vi "Mini_Test_App.vi"() -> ()   [LabVIEW 2015]
uses:
  Type Definitions/Mini_Test_App_Data.ctl
  <vilib>/Utility/error.llb/DialogType.ctl
panel:
  out "HP FAIL":bool
  out "HP PASS":bool
  out "HP UT":bool
  in  "Stop Hi-Pot":bool
  in  "Start Hi-Pot":bool
  out "GB FAIL":bool
  out "GB PASS":bool
  out "GB UT":bool
  in  "Stop GB":bool
  in  "Start GB":bool
  in  "Exit":bool
  # "Interface type: NI USB-6525"
  # "Warning. This app is a proof of concept and has no other purpose, \nit is not intended for production. Likewise, it has no error handling. \nUse at your own risk."
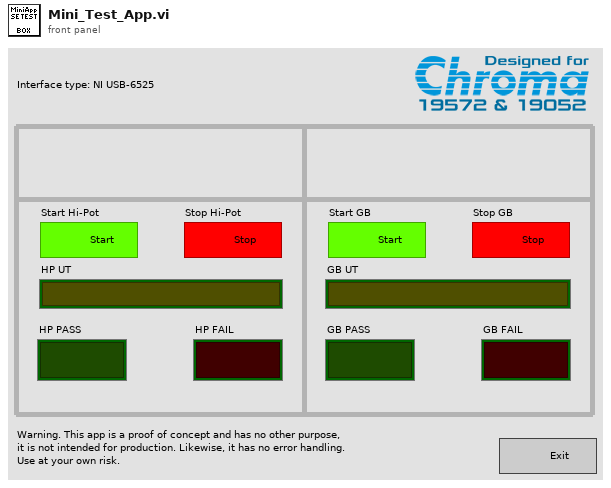
[diagram p1: front panel]
types:
  T1 = typedef "DialogType.ctl" = u16
  T2 = typedef "Mini_Test_App_Data.ctl" = cluster{"GB states":cluster{"UT":bool, "PASS":bool, "FAIL":bool}, "HP states":cluster{"UT":bool, "PASS":bool, "FAIL":bool}}
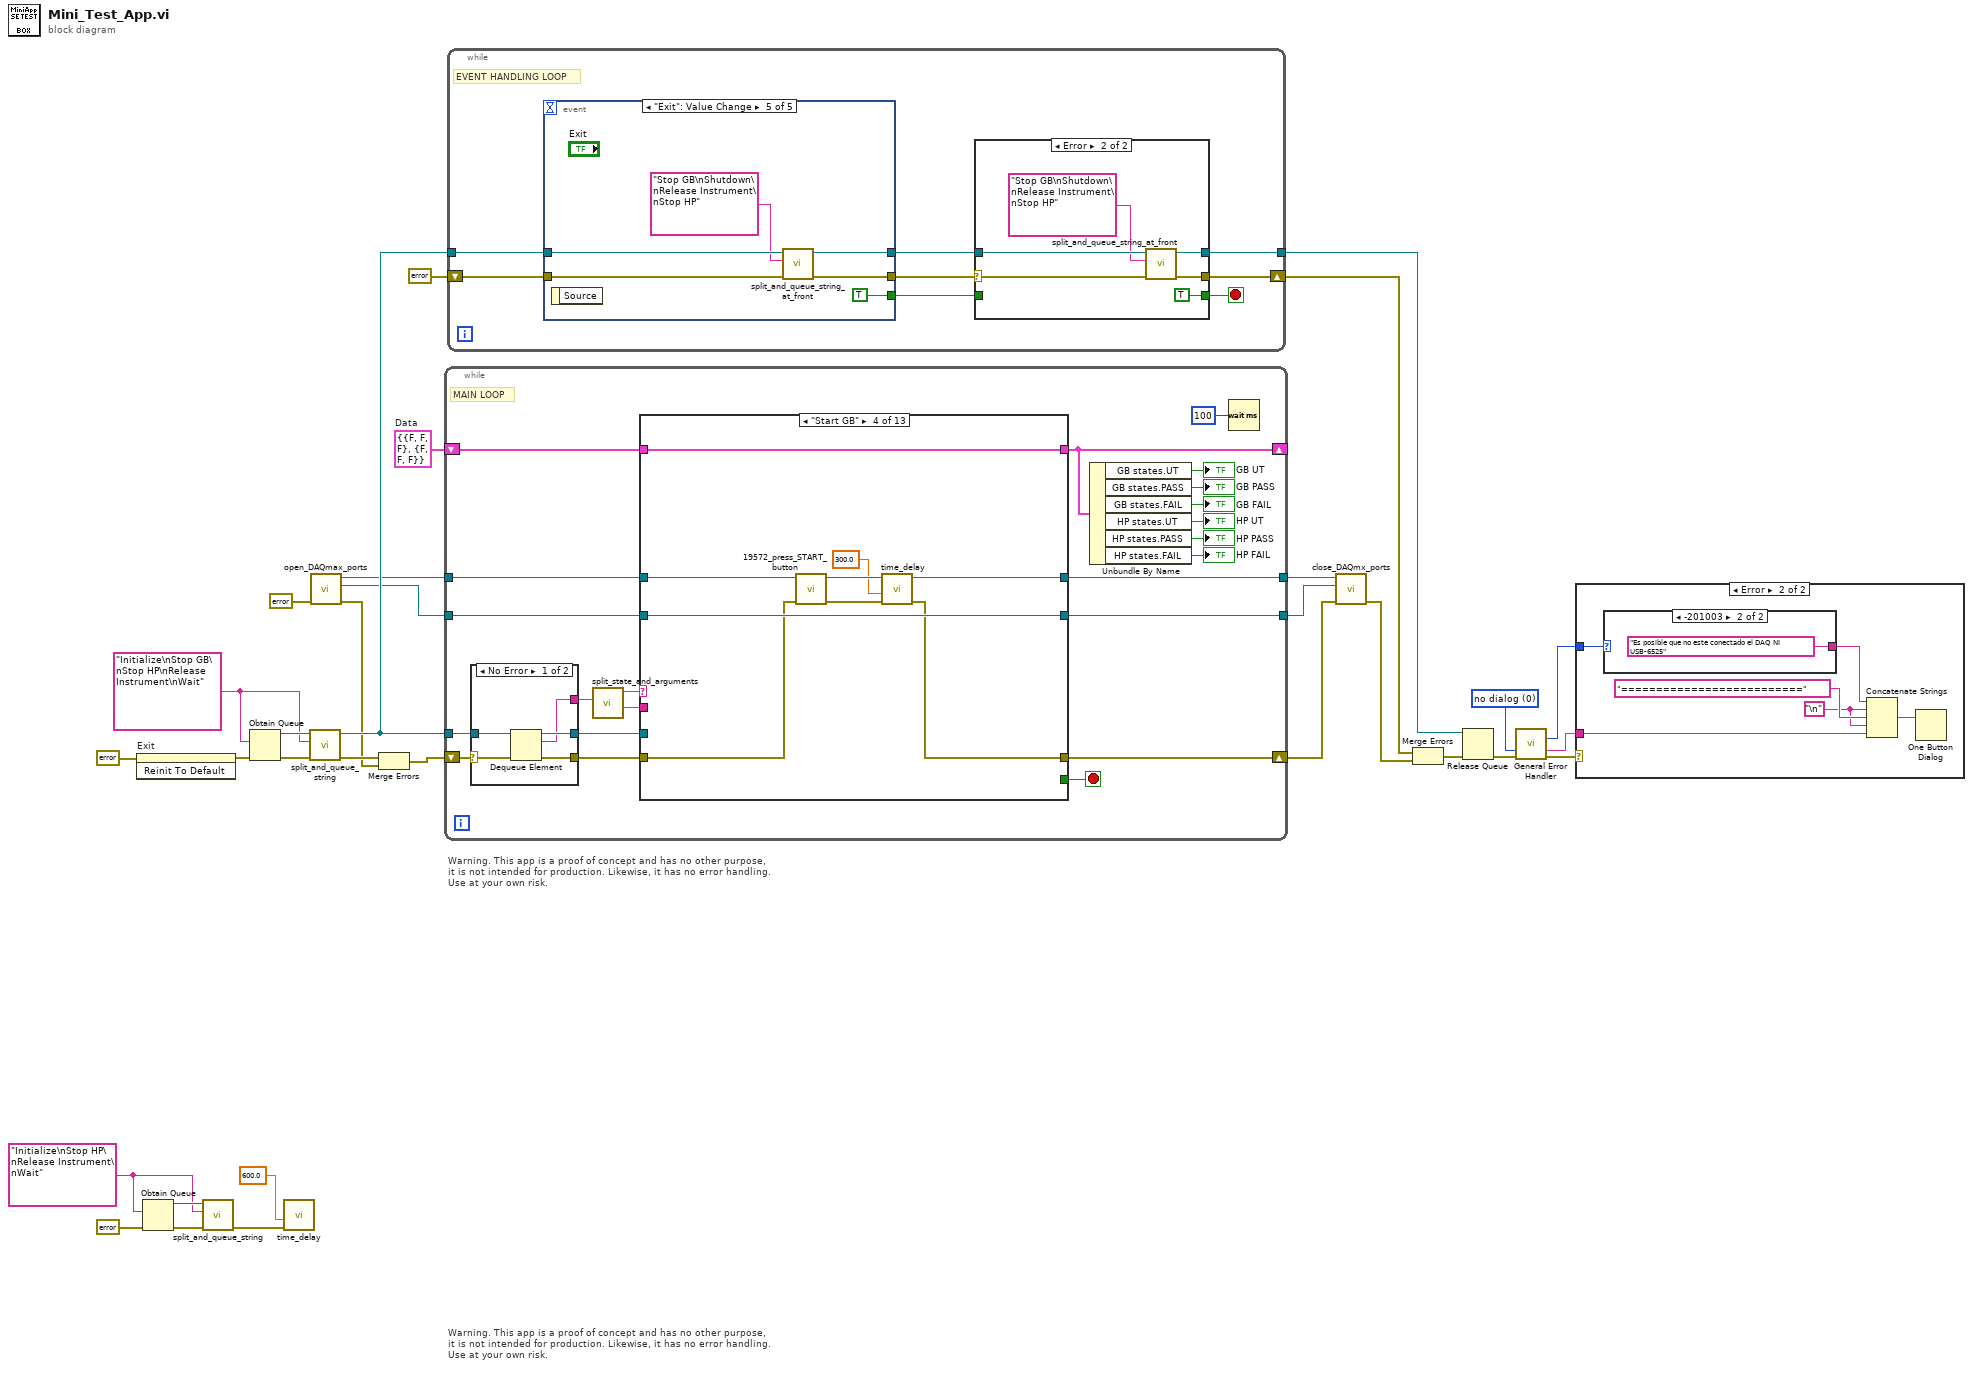
[diagram p0: block diagram]
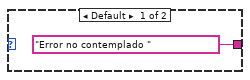
[diagram p3: hidden frame]
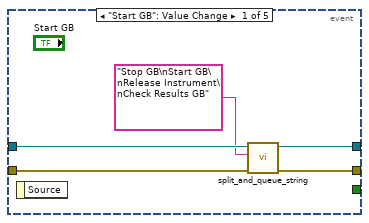
[diagram p5: hidden frame]
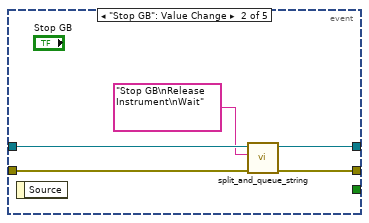
[diagram p6: hidden frame]
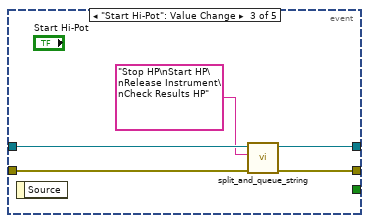
[diagram p7: hidden frame]
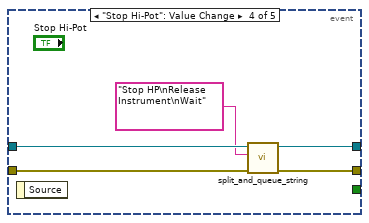
[diagram p8: hidden frame]
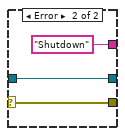
[diagram p9: hidden frame]
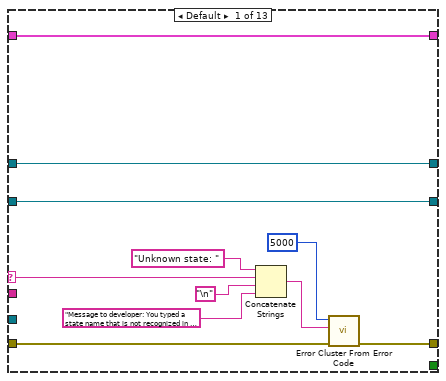
[diagram p10: hidden frame]
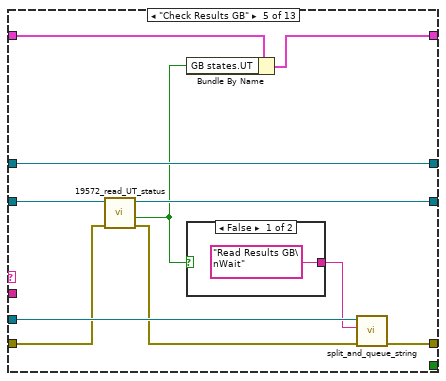
[diagram p13: hidden frame]
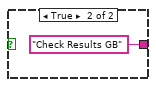
[diagram p14: hidden frame]
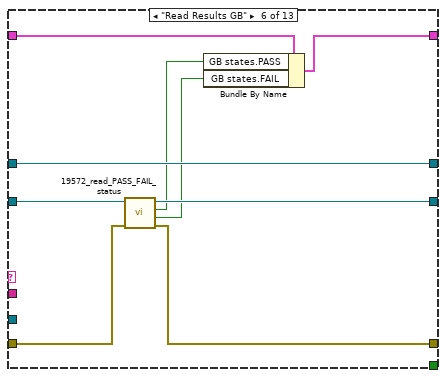
[diagram p15: hidden frame]
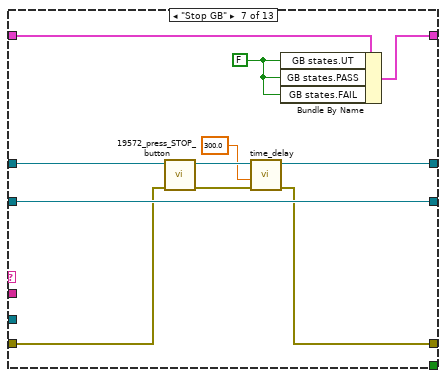
[diagram p16: hidden frame]
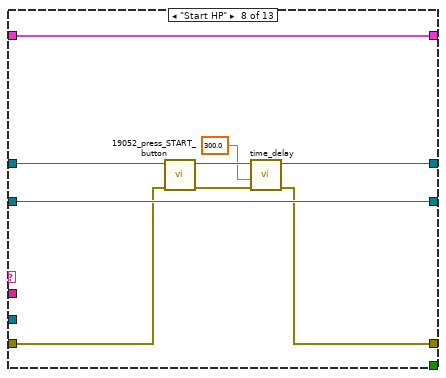
[diagram p17: hidden frame]
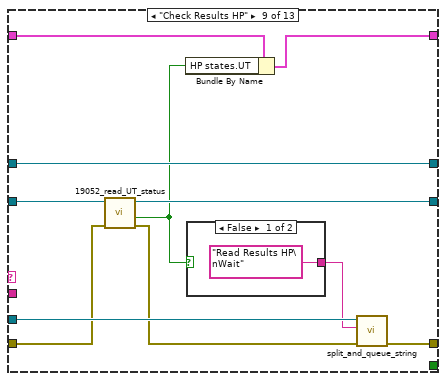
[diagram p18: hidden frame]
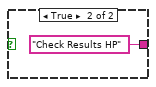
[diagram p19: hidden frame]
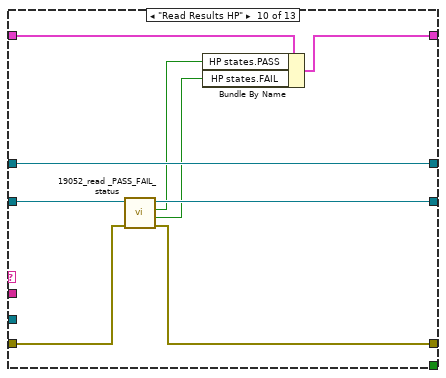
[diagram p20: hidden frame]
diagram:
  w1 = T1 0 items=["no dialog", "OK message", "continue or stop message", "OK message + warnings", "continue/stop + warnings"] ("type of dialog (OK msg:1)")
  w11 = "Initialize\nStop HP\nRelease Instrument\nWait"
  w20 = T2 {"GB states"={"UT"=FALSE, "PASS"=FALSE, "FAIL"=FALSE}, "HP states"={"UT"=FALSE, "PASS"=FALSE, "FAIL"=FALSE}}  # Data
  w22 = "Initialize\nStop GB\nStop HP\nRelease Instrument\nWait"
  # "Warning. This app is a proof of concept and has no other purpose, \nit is not intended for production. Likewise, it has no error handling. \nUse at your own risk."
  # "Warning. This app is a proof of concept and has no other purpose, \nit is not intended for production. Likewise, it has no error handling. \nUse at your own risk."
  n1 = invoke on="Exit" class="Bool (strict)" method="Reinit To Default"(error in=errorcluster {"status"=FALSE, "code"=0, "source"=""} ("error constant")) -> (error out=w17:errorcluster)  [unwired: 2 in, 2 out]
  n2 = Obtain Queue(element data type=w11, error in (no error)=errorcluster {"status"=FALSE, "code"=0, "source"=""} ("error constant")) -> (queue out=w13:refnum<queue>, error out=w12:errorcluster)  [unwired: 3 in, 1 out]
  n3 = call "split_and_queue_string.vi"("error in (no error)"=w12, "program string"=w11, "queue in"=w13) -> ("error out"=w7:errorcluster)  [unwired: 7 in, 1 out]
  n4 = Obtain Queue(element data type=w22, error in (no error)=w17) -> (queue out=w26:refnum<queue>, error out=w28:errorcluster)  [unwired: 3 in, 1 out]
  n5 = call "time_delay.vi"("error in (no error)"=w7, "milliseconds to wait"=600.0) -> ()  [unwired: 9 in, 1 out]
  n6 = call "split_and_queue_string.vi"("error in (no error)"=w28, "program string"=w22, "queue in"=w26) -> ("error out"=w27:errorcluster, "queue out"=w32:refnum<queue>)  [unwired: 7 in]
  n7 = call "open_DAQmax_ports.vi"("error in (no error)"=errorcluster {"status"=FALSE, "code"=0, "source"=""} ("error constant")) -> ("error out"=w21:errorcluster, "UT/PASS/FAIL states out"=w14:refnum<k21>, "START/STOP buttons out"=w15:refnum<k21>)  [unwired: 8 in]
  n8 = Merge Errors(w27, w21) -> (w16:errorcluster)
  n9 = while {
    tunnel: w15 -> [w49]
    tunnel: w14 -> [w48]
    shift-right: [w53] -> w23
    shift-left: w16 -> [w52]
    tunnel: [w50] -> w30
    tunnel: [w47] -> w29
    tunnel: w32 -> [w45]
    shift-right: [w39] -> _
    shift-left: w20 -> [w40]
    stop <- w46 stop-if-true
    # "MAIN LOOP"
    n10 = case shown="No Error" w52 {
      selector: w52 -> [w58 w61]
      tunnel: [w57 w61] -> w51
      tunnel: w45 -> [w59 w62]
      tunnel: [w56 w62] -> w44
      tunnel: [w55 "Shutdown"] -> w41
      frame No Error {
        n11 = Dequeue Element(queue=w59, error in (no error)=w58) -> (queue out=w56:refnum<queue>, element=w55:string, error out=w57:errorcluster)  [unwired: 1 in, 1 out]
      }
      frame Error {
      }
    }
    n12 = call "split_state_and_arguments.vi"("String"=w41) -> ("Arguments"=w42:string, "State"=w43:string)  [unwired: 9 in]
    n13 = case shown="\"Start GB\"" w43 {
      selector: w43 -> [w65 _ _ _ _ _ _ _ _ _ _ _ _]
      tunnel: [w67 w77 w81 w83 w93 w104 w112 w122 w135 w148 w155 w162 w173] -> w53
      tunnel: w51 -> [w66 w77 w81 w86 w96 w108 w118 w123 w137 w149 w156 w163 w174]
      tunnel: [w73 w76 w80 w87 w99 w111 w119 w125 w140 w151 w161 w164 w171] -> w50
      tunnel: w49 -> [w73 w76 w80 w88 w99 w111 w120 w126 w140 w151 w157 w165 w171]
      tunnel: w48 -> [w72 w75 w79 w89 w98 w110 w121 w129 w138 w150 w160 w167 w170]
      tunnel: [w72 w75 w79 w89 w97 w109 w121 w129 w133 w147 w160 w167 w170] -> w47
      tunnel: [_ _ _ _ _ _ _ _ _ _ _ _ w172] -> w46
      tunnel: w44 -> [_ _ _ _ w100 _ _ _ w139 _ _ _ _]
      tunnel: w42 -> [_ _ _ _ _ _ _ _ _ _ _ _ _]
      tunnel: [w64 w74 w78 w82 w95 w103 w116 w128 w131 w145 w152 w166 w169] -> w39
      tunnel: w40 -> [w64 w74 w78 w82 w91 w107 w117 w128 w132 w146 w153 w166 w169]
      frame Default {
        n14 = Concatenate Strings("Unknown state: " ("string"), w65, "\n", "Message to developer: You typed a state name that is not recognized in gb test loop.") -> (w70:string)
        n15 = call <vilib>:"Error Cluster From Error Code.vi"("error in (no error)"=w66, "error message (\"\")"=w70, "error code (0)"=5000) -> ("error out"=w67:errorcluster)  [unwired: 6 in]
      }
      frame "Initialize" {
      }
      frame "Wait" {
      }
      frame "Start GB" {
        n16 = call "19572_press_START_button.vi"("error in (no error)"=w86, "task/channels in"=w88) -> ("error out"=w85:errorcluster, "task out"=w87:refnum<k21>)  [unwired: 8 in]
        n17 = call "time_delay.vi"("error in (no error)"=w85, "milliseconds to wait"=300.0) -> ("error out"=w83:errorcluster)  [unwired: 9 in]
      }
      frame "Check Results GB" {
        n18 = call "19572_read_UT_status.vi"("error in (no error)"=w96, "task/channles in"=w98) -> ("error out"=w94:errorcluster, "Under Test"=w90:bool, "task out"=w97:refnum<k21>)  [unwired: 7 in]
        n19 = Bundle By Name(cluster=w91, "GB states.UT"=w90) -> (w95:T2)
        n20 = case shown="False" w90 {
          tunnel: ["Read Results GB\nWait" "Check Results GB"] -> w92
          frame False {
          }
          frame True {
          }
        }
        n21 = call "split_and_queue_string.vi"("error in (no error)"=w94, "program string"=w92, "queue in"=w100) -> ("error out"=w93:errorcluster)  [unwired: 7 in, 1 out]
      }
      frame "Read Results GB" {
        n22 = call "19572_read_PASS_FAIL_status.vi"("error in (no error)"=w108, "task/channels in"=w110) -> ("error out"=w104:errorcluster, "Fail"=w106:bool, "Pass"=w105:bool, "task out"=w109:refnum<k21>)  [unwired: 6 in]
        n23 = Bundle By Name(cluster=w107, "GB states.PASS"=w105, "GB states.FAIL"=w106) -> (w103:T2)
      }
      frame "Stop GB" {
        w113 = FALSE
        n24 = call "19572_press_STOP_button.vi"("error in (no error)"=w118, "task/channels in"=w120) -> ("error out"=w115:errorcluster, "task out"=w119:refnum<k21>)  [unwired: 8 in]
        n25 = call "time_delay.vi"("error in (no error)"=w115, "milliseconds to wait"=300.0) -> ("error out"=w112:errorcluster)  [unwired: 9 in]
        n26 = Bundle By Name(cluster=w117, "GB states.UT"=w113, "GB states.PASS"=w113, "GB states.FAIL"=w113) -> (w116:T2)
      }
      frame "Start HP" {
        n27 = call "19052_press_START_button.vi"("error in (no error)"=w123, "task/channels in"=w126) -> ("error out"=w127:errorcluster, "task out"=w125:refnum<k21>)  [unwired: 8 in]
        n28 = call "time_delay.vi"("error in (no error)"=w127, "milliseconds to wait"=300.0) -> ("error out"=w122:errorcluster)  [unwired: 9 in]
      }
      frame "Check Results HP" {
        n29 = call "19052_read_UT_status.vi"("error in (no error)"=w137, "task/channels in"=w138) -> ("error out"=w136:errorcluster, "Under  Test"=w130:bool, "task out"=w133:refnum<k21>)  [unwired: 7 in]
        n30 = Bundle By Name(cluster=w132, "HP states.UT"=w130) -> (w131:T2)
        n31 = case shown="False" w130 {
          tunnel: ["Read Results HP\nWait" "Check Results HP"] -> w134
          frame False {
          }
          frame True {
          }
        }
        n32 = call "split_and_queue_string.vi"("error in (no error)"=w136, "program string"=w134, "queue in"=w139) -> ("error out"=w135:errorcluster)  [unwired: 7 in, 1 out]
      }
      frame "Read Results HP" {
        n33 = call "19052_read _PASS_FAIL_status.vi"("error in (no error)"=w149, "task/channels in"=w150) -> ("error out"=w148:errorcluster, "Fail"=w143:bool, "Pass"=w144:bool, "task out"=w147:refnum<k21>)  [unwired: 6 in]
        n34 = Bundle By Name(cluster=w146, "HP states.PASS"=w144, "HP states.FAIL"=w143) -> (w145:T2)
      }
      frame "Stop HP" {
        w154 = FALSE
        n35 = call "19052_press_STOP_button.vi"("error in (no error)"=w156, "task/channels in"=w157) -> ("error out"=w158:errorcluster, "task out"=w161:refnum<k21>)  [unwired: 8 in]
        n36 = call "time_delay.vi"("error in (no error)"=w158, "milliseconds to wait"=300.0) -> ("error out"=w155:errorcluster)  [unwired: 9 in]
        n37 = Bundle By Name(cluster=w153, "HP states.UT"=w154, "HP states.PASS"=w154, "HP states.FAIL"=w154) -> (w152:T2)
      }
      frame "Release Instrument" {
        n38 = call "19XX2_release_ALL.vi"("error in (no error)"=w163, "Refnum in"=w165) -> ("error out"=w162:errorcluster, "Refnum out"=w164:refnum<k21>)  [unwired: 8 in]
      }
      frame "Shutdown" {
        w172 = TRUE
        n39 = property on="Exit" class="Bool (strict)"("Val(Sgnl)"=w172) -> (error out=w168:errorcluster)  [unwired: 2 in, 1 out]
        n40 = Merge Errors(w174, w168) -> (w173:errorcluster)
      }
    }
    n41 = Unbundle By Name(w39) -> ("GB states.UT"=→"GB UT":bool, "GB states.PASS"=→"GB PASS":bool, "GB states.FAIL"=→"GB FAIL":bool, "HP states.UT"=→"HP UT":bool, "HP states.PASS"=→"HP PASS":bool, "HP states.FAIL"=→"HP FAIL":bool)
    n42 = Wait (ms)(milliseconds to wait=u32 100) -> ()  [unwired: 1 out]
  }
  n43 = while {
    shift-right: [w177] -> w18
    shift-left: errorcluster {"status"=FALSE, "code"=0, "source"=""} ("error constant") -> [w182]
    tunnel: w32 -> [w181]
    tunnel: [w179] -> w25
    stop <- w175 stop-if-true
    # "EVENT HANDLING LOOP"
    n44 = event shown="[4] \"Exit\": Value Change" {
      selector: _ -> [_ _ _ _ _]
      dyn-events: _ -> [_ _ _ _ _]
      timeout: _ -> [_ _ _ _ _]
      tunnel: [w196 w200 w205 w210 w212] -> w178
      tunnel: w182 -> [w192 w201 w206 w211 w217]
      tunnel: w181 -> [w195 w199 w204 w209 w216]
      tunnel: [w194 w198 w203 w208 w215] -> w180
      tunnel: [_ _ _ _ TRUE] -> w176
      event "Start GB": Value Change {
        n45 = event-data() -> ()  [unwired: 1 in, 1 out]
        n46 = call "split_and_queue_string.vi"("error in (no error)"=w192, "program string"="Stop GB\nStart GB\nRelease Instrument\nCheck Results GB", "queue in"=w195) -> ("error out"=w196:errorcluster, "queue out"=w194:refnum<queue>)  [unwired: 7 in]
      }
      event "Stop GB": Value Change {
        n47 = event-data() -> ()  [unwired: 1 in, 1 out]
        n48 = call "split_and_queue_string.vi"("error in (no error)"=w201, "program string"="Stop GB\nRelease Instrument\nWait", "queue in"=w199) -> ("error out"=w200:errorcluster, "queue out"=w198:refnum<queue>)  [unwired: 7 in]
      }
      event "Start Hi-Pot": Value Change {
        n49 = event-data() -> ()  [unwired: 1 in, 1 out]
        n50 = call "split_and_queue_string.vi"("error in (no error)"=w206, "program string"="Stop HP\nStart HP\nRelease Instrument\nCheck Results HP", "queue in"=w204) -> ("error out"=w205:errorcluster, "queue out"=w203:refnum<queue>)  [unwired: 7 in]
      }
      event "Stop Hi-Pot": Value Change {
        n51 = event-data() -> ()  [unwired: 1 in, 1 out]
        n52 = call "split_and_queue_string.vi"("error in (no error)"=w211, "program string"="Stop HP\nRelease Instrument\nWait", "queue in"=w209) -> ("error out"=w210:errorcluster, "queue out"=w208:refnum<queue>)  [unwired: 7 in]
      }
      event "Exit": Value Change {
        n53 = event-data() -> ()  [unwired: 1 in, 1 out]
        n54 = call "split_and_queue_string_at_front.vi"("error in (no error)"=w217, "program string"="Stop GB\nShutdown\nRelease Instrument\nStop HP", "queue in"=w216) -> ("error out"=w212:errorcluster, "queue out"=w215:refnum<queue>)  [unwired: 7 in]
      }
    }
    n55 = case shown="Error" w178 {
      selector: w178 -> [w184 w189]
      tunnel: w180 -> [w185 w191]
      tunnel: [w185 w190] -> w179
      tunnel: [w184 w187] -> w177
      tunnel: w176 -> [w183 _]
      tunnel: [w183 TRUE] -> w175
      frame No Error {
      }
      frame Error {
        n56 = call "split_and_queue_string_at_front.vi"("error in (no error)"=w189, "program string"="Stop GB\nShutdown\nRelease Instrument\nStop HP", "queue in"=w191) -> ("error out"=w187:errorcluster, "queue out"=w190:refnum<queue>)  [unwired: 7 in]
      }
    }
  }
  n57 = call "close_DAQmx_ports.vi"("error in (no error)"=w23, "task/channels in 2"=w29, "task/channels in 1"=w30) -> ("error out"=w24:errorcluster)  [unwired: 8 in]
  n58 = Merge Errors(w18, w24) -> (w19:errorcluster)
  n59 = Release Queue(queue=w25, error in (no error)=w19) -> (error out=w8:errorcluster)  [unwired: 1 in, 2 out]
  n60 = call <vilib>:"General Error Handler.vi"("type of dialog (OK msg:1)"=w1, "error in (no error)"=w8) -> ("code out"=w2:i32, "message"=w3:string, "error out"=w4:errorcluster)  [unwired: 9 in, 2 out]
  n61 = case shown="Error" w4 {
    tunnel: w2 -> [_ w223]
    tunnel: w3 -> [_ w221]
    frame No Error {
    }
    frame Error {
      w218 = "\n"
      n62 = case shown="-201003" w223 {
        tunnel: ["Error no contemplado " "Es posible que no este conectado el DAQ NI USB-6525"] -> w222
        frame Default {
        }
        frame -201003 {
        }
      }
      n63 = Concatenate Strings(w222, w218, "==========================", w218, w221) -> (w220:string)
      n64 = One Button Dialog(message=w220) -> ()  [unwired: 1 in, 1 out]
    }
  }
